vi "ALS_Prepend Time Stamp To Data File in Path.vi"(8 "error in (no error)":errorcluster, 11 "Data Log Path":path=path "C:/ALS-321 Release Tester/Log_Files/Data Log.txt") -> (0 "error out":errorcluster, 3 "Data Log Path Out":path=path "C:/ALS-321 Release Tester/Log_Files/Data Log.txt")   [LabVIEW 2010]
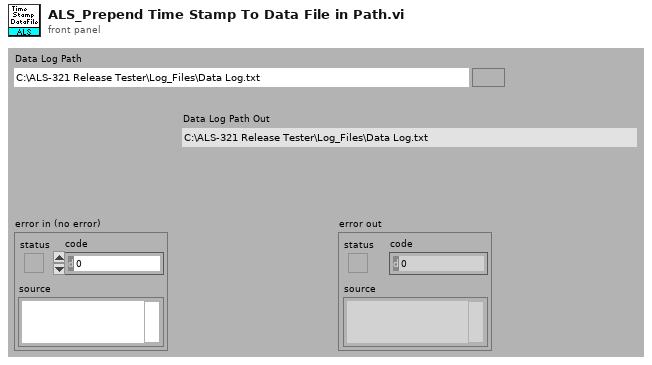
[diagram p1: front panel]
types:
  T1 = typedef "LVDateTimeRec.ctl" = cluster{"fractional second":dbl, "second":i32, "minute":i32, "hour":i32, "day of month":i32, "month":i32, "year":i32, "day of week":i32, "day of year":i32, "DST":i32}
  T2 = cluster{"fractional second":string, "second":string, "minute":string, "hour":string, "day of month":string, "month":string, "year":string, "day of week":string, "day of year":string, "DST":string}
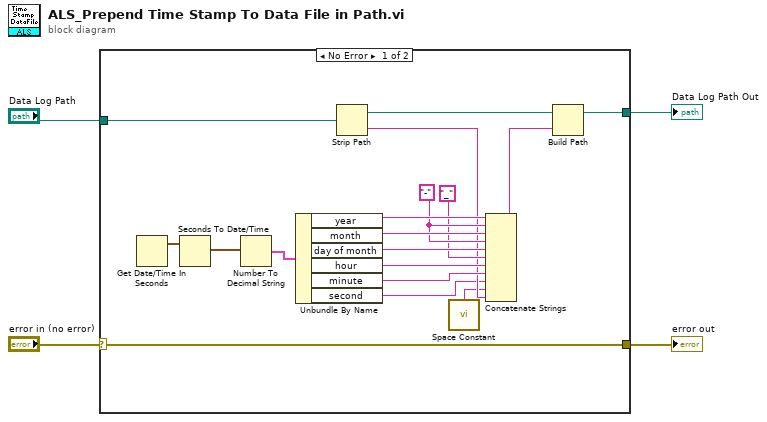
[diagram p0: block diagram]
diagram:
  n1 = case shown="No Error" "error in (no error)" {
    selector: "error in (no error)" -> [w8 w23]
    tunnel: "Data Log Path" -> [w22 w24]
    tunnel: [w20 w24] -> w3
    tunnel: [w8 w23] -> w1
    frame No Error {
      w14 = "-" ("new character")
      n2 = Get Date/Time In Seconds() -> (seconds since 1Jan1904=w19:timestamp)
      n3 = Seconds To Date/Time(time stamp (now)=w19) -> (date time rec=w18:T1)  [unwired: 1 in]
      n4 = Number To Decimal String(number=w18) -> (decimal integer string=w17:T2)  [unwired: 1 in]
      n5 = Unbundle By Name(w17) -> ("year"=w16:string, "month"=w15:string, "day of month"=w13:string, "hour"=w11:string, "minute"=w10:string, "second"=w5:string)
      n6 = Strip Path(path=w22) -> (stripped path=w21:path, name=w7:string)
      n7 = call <vilib>:"Space Constant.vi"() -> ("String"=w6:string)
      n8 = Concatenate Strings(w16, w14, w15, w14, w13, "_", w11, w10, w5, w6, w7) -> (w9:string)
      n9 = Build Path(base path=w21, name or relative path=w9) -> (appended path=w20:path)
    }
    frame Error {
    }
  }
  "Data Log Path Out" <- w3
  "error out" <- w1
